vi "Time to Day-Hr-Min-Sec-msec.vi"(2 "Time in millisec":dbl format="%#.1f") -> (7 "Time Day/Hr:Min:Sec:msec":string)   [LabVIEW 2020]
doc: "Converts time in milliseconds to string Day/Hr:Min:Sec.msec"
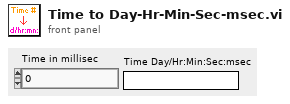
[diagram p1: front panel]
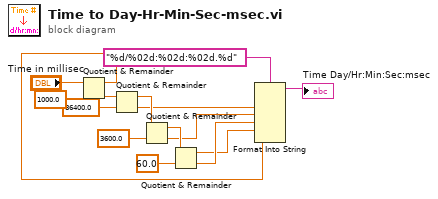
[diagram p0: block diagram]
diagram:
  n1 = Quotient & Remainder(x="Time in millisec", y=1000.0) -> (x-y*floor(x/y)=w3:dbl, floor(x/y)=w13:dbl)
  n2 = Quotient & Remainder(x=w13, y=86400.0) -> (x-y*floor(x/y)=w11:dbl, floor(x/y)=w7:dbl)
  n3 = Quotient & Remainder(x=w11, y=3600.0) -> (x-y*floor(x/y)=w9:dbl, floor(x/y)=w6:dbl)
  n4 = Quotient & Remainder(x=w9, y=60.0) -> (x-y*floor(x/y)=w4:dbl, floor(x/y)=w5:dbl)
  n5 = Format Into String(format string="%d/%02d:%02d:%02d.%d", w7, w6, w5, w4, w3) -> (resulting string=→"Time Day/Hr:Min:Sec:msec":string)  [unwired: 2 in, 1 out]
